vi "Evaluate Match.vi"(7 "Topic":string, 8 "error in (no error)":errorcluster, 11 "Subscription in":refnum<class "Subscription.lvclass">) -> (0 "error out":errorcluster, 1 "Cached?":bool, 2 "Matched":bool, 3 "Subscription out":refnum<class "Subscription.lvclass">)   [LabVIEW 2013, in "MQTT Base.lvlib" / "Subscription.lvclass"]
uses:
  Subscription.lvclass
  Subscription.lvclass/Subscription.ctl
  TopicFilter/TopicFilter.lvclass/TopicFilter.ctl
  TopicFilter/TopicFilter.lvclass
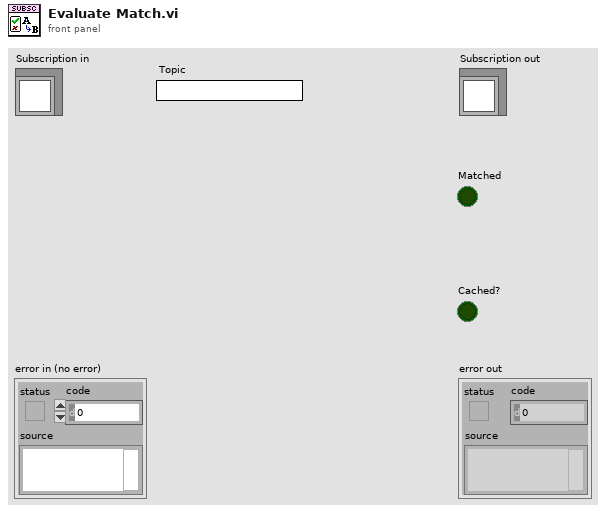
[diagram p1: front panel]
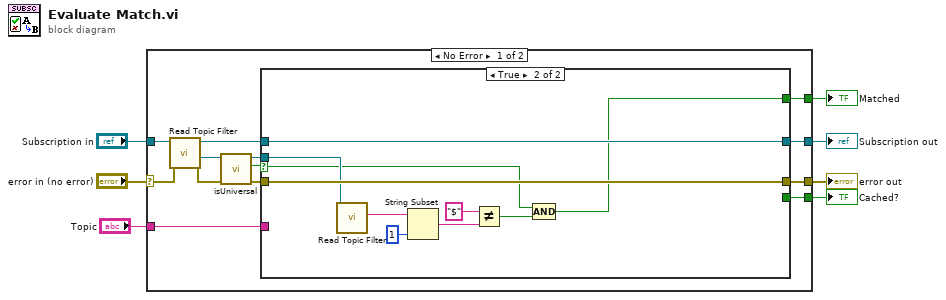
[diagram p0: block diagram]
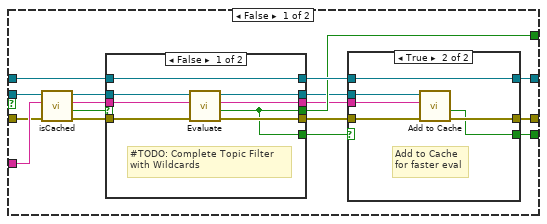
[diagram p2: hidden frame]
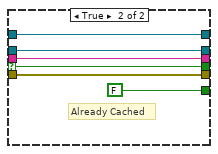
[diagram p4: hidden frame]
diagram:
  n1 = case shown="No Error" "error in (no error)" {
    selector: "error in (no error)" -> [w17 w71]
    tunnel: [w14 w71] -> w6
    tunnel: [w13 w70] -> w4
    tunnel: "Subscription in" -> [w19 w70]
    tunnel: "Topic" -> [w18 _]
    tunnel: [w11 _] -> w2
    tunnel: [w12 _] -> w1
    frame No Error {
      n2 = call "Read Topic Filter.vi"("error in (no error)"=w17, "Subscription in"=w19) -> ("error out"=w16:errorcluster, "Instance"=w10:refnum<class "TopicFilter.lvclass">, "Subscription out"=w15:refnum<class "Subscription.lvclass">)  [unwired: 6 in, 1 out]
      n3 = call "isUniversal.vi"("TopicFilter in"=w10) -> ("universal"=w8:bool, "TopicFilter out"=w9:refnum<class "TopicFilter.lvclass">)  [unwired: 9 in]
      n4 = case shown="True" w8 {
        selector: w8 -> [_ w61]
        tunnel: w18 -> [w36 _]
        tunnel: w16 -> [w32 w68]
        tunnel: w15 -> [w31 w69]
        tunnel: [w28 w68] -> w14
        tunnel: [w27 w69] -> w13
        tunnel: [w24 _] -> w12
        tunnel: [w23 w60] -> w11
        tunnel: w9 -> [w20 w67]
        frame False {
          n5 = call "isCached.vi"("error in (no error)"=w32, "Topic"=w36, "TopicFilter in"=w20) -> ("error out"=w33:errorcluster, "found?"=w30:bool, "Topic dup"=w34:string, "TopicFilter out"=w35:refnum<class "TopicFilter.lvclass">)  [unwired: 5 in]
          n6 = case shown="False" w30 {
            selector: w30 -> [_ w57]
            tunnel: w35 -> [w53 w54]
            tunnel: w34 -> [w52 w55]
            tunnel: [w48 w57] -> w23
            tunnel: w33 -> [w51 w58]
            tunnel: [w50 w58] -> w29
            tunnel: w31 -> [w49 w59]
            tunnel: [w49 w59] -> w26
            tunnel: [w48 FALSE] -> w25
            tunnel: [w47 w55] -> w22
            tunnel: [w46 w54] -> w21
            frame False {
              # "#TODO: Complete Topic Filter\nwith Wildcards"
              n7 = call "Evaluate.vi"("error in (no error)"=w51, "Topic"=w52, "TopicFilter in"=w53) -> ("error out"=w50:errorcluster, "Match"=w48:bool, "Topic dup"=w47:string, "TopicFilter out"=w46:refnum<class "TopicFilter.lvclass">)  [unwired: 5 in]
            }
            frame True {
              # "Already Cached"
            }
          }
          n8 = case shown="True" w25 {
            selector: w25 -> [w39 _]
            tunnel: w29 -> [w37 w42]
            tunnel: [w37 w41] -> w28
            tunnel: w26 -> [w38 w45]
            tunnel: [w38 w45] -> w27
            tunnel: [w39 w40] -> w24
            tunnel: w22 -> [_ w43]
            tunnel: w21 -> [_ w44]
            frame False {
            }
            frame True {
              # "Add to Cache\nfor faster eval"
              n9 = call "Add to Cache.vi"("error in (no error)"=w42, "Topic"=w43, "TopicFilter in"=w44) -> ("error out"=w41:errorcluster, "added to cache"=w40:bool)  [unwired: 6 in, 1 out]
            }
          }
        }
        frame True {
          n10 = call "Read Topic Filter.vi"("TopicFilter in"=w67) -> ("Topic Filter"=w66:string)  [unwired: 9 in, 1 out]
          n11 = String Subset(string=w66, length (rest)=1 ("length (rest)")) -> (substring=w64:string)  [unwired: 1 in]
          n12 = Not Equal?(x="$", y=w64) -> (x != y?=w62:bool)
          n13 = Compound Arithmetic op=AND(w61, w62) -> (w60:bool)
        }
      }
    }
    frame Error {
    }
  }
  "error out" <- w6
  "Subscription out" <- w4
  "Matched" <- w2
  "Cached?" <- w1
